vi "Replay AVI Movie.vi"() -> ()   [LabVIEW 2015]
panel:
  in  "Bin Iteration":i32
  in  "Frame Interval (ms)":u32=100
  in  "AVI File Name":path=path "Z:/1_20140213R_Edited.avi"
  in  "N Frame":i32=100
  out "Frame #":i32
  out "Bin Image":T1(plugin-control)
  out "Original Image":T1(plugin-control)
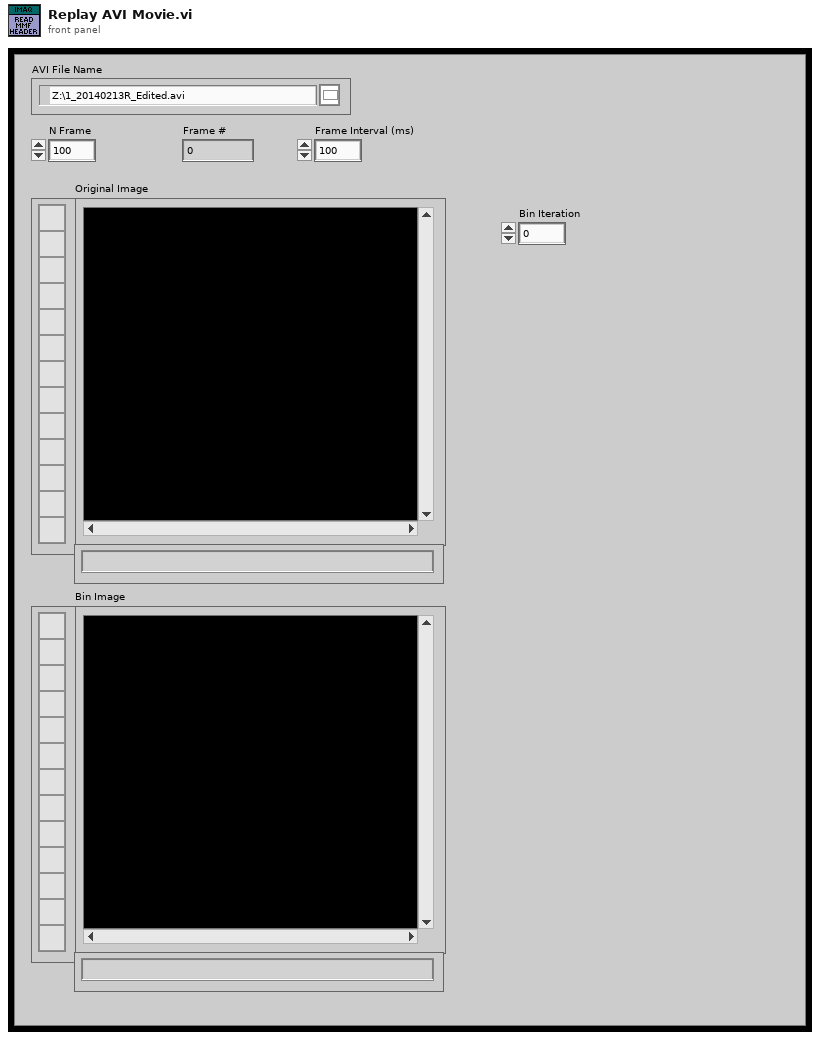
[diagram p1: front panel]
types:
  T1 = typedef "IMAQ Image.ctl" = refnum<image>
  T2 = typedef "IMAQ AVI2 Refnum.ctl" = refnum<k20>
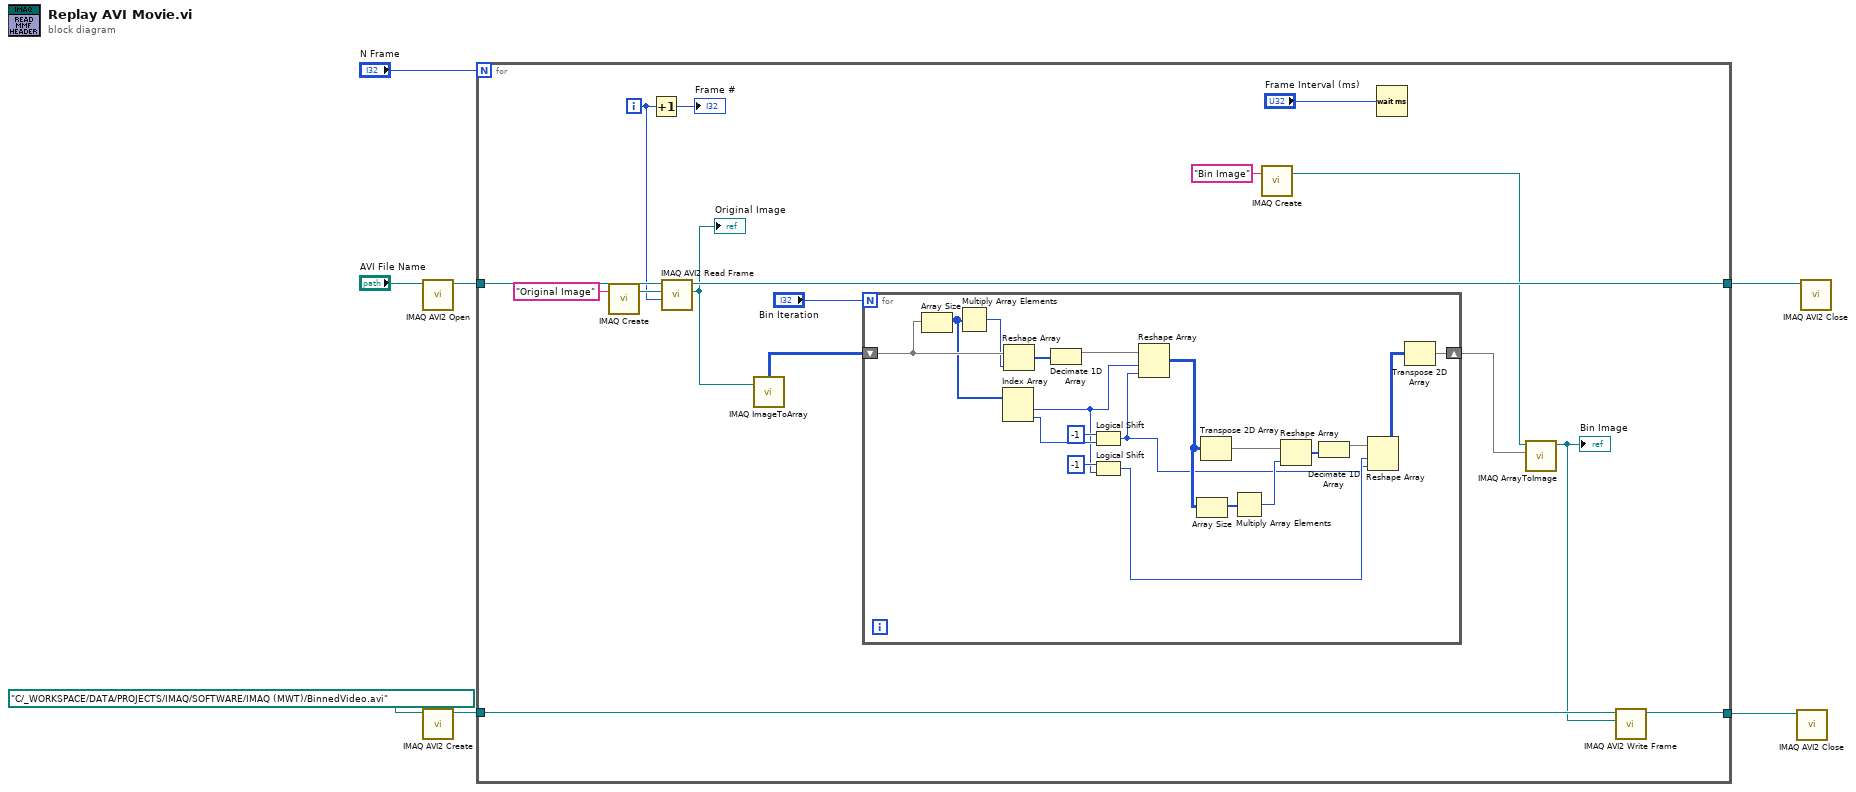
[diagram p0: block diagram]
diagram:
  n1 = call "IMAQ AVI2 Open"("AVI File Path"="AVI File Name") -> ("AVI Refnum"=w4:T2)  [unwired: 9 in, 1 out]
  n2 = call "IMAQ AVI2 Create"("AVI Path"=path "C:/_WORKSPACE/DATA/PROJECTS/IMAQ/SOFTWARE/IMAQ (MWT)/BinnedVideo.avi" ("AVI File Path")) -> ("AVI Refnum"=w2:T2)  [unwired: 9 in, 1 out]
  n3 = for {
    N: "N Frame" -> [_]
    tunnel: w4 -> [w22]
    tunnel: [w21] -> w7
    tunnel: w2 -> [w10]
    tunnel: [w9] -> w1
    i -> [w12]
    n4 = call "IMAQ Create"("Image Name"="Original Image") -> ("New Image"=w13:T1)  [unwired: 4 in, 1 out]
    n5 = Increment(x=w12) -> (x+1=→"Frame #":i32)
    n6 = call "IMAQ AVI2 Read Frame"("Frame Number"=w12, "Image"=w13, "AVI Refnum"=w22) -> ("Image Out"=w18:T1, "AVI Refnum (duplicate)"=w21:T2)  [unwired: 6 in, 1 out]
    "Original Image" <- w18
    n7 = call "IMAQ ImageToArray"("Image"=w18) -> ("Image Pixels (U8)"=w17:u8[][])  [unwired: 3 in, 4 out]
    n8 = for {
      N: "Bin Iteration" -> [_]
      shift-right: [w24] -> w16
      shift-left: w17 -> [w42]
      n9 = Array Size(array=w42) -> (size(s)=w39:i32[])
      n10 = Multiply Array Elements(1:w39) -> (0:w41:i32)
      n11 = Index Array(array=w39) -> (element #1=w30:i32, element #2=w38:i32)  [unwired: 2 in]
      n12 = Reshape Array(w42, w41) -> (w40:u8[])
      n13 = Decimate 1D Array(w40) -> (w26:u8[])  [unwired: 1 out]
      n14 = Logical Shift(y=i16 -1, x=w38) -> (x << y=w28:i32)
      n15 = Logical Shift(y=i16 -1, x=w30) -> (x << y=w29:i32)
      n16 = Reshape Array(w26, w30, w28) -> (w34:u8[][])
      n17 = Array Size(array=w34) -> (size(s)=w35:i32[])
      n18 = Transpose 2D Array(2D array=w34) -> (transposed array=w36:u8[][])
      n19 = Multiply Array Elements(1:w35) -> (0:w33:i32)
      n20 = Reshape Array(w36, w33) -> (w32:u8[])
      n21 = Decimate 1D Array(w32) -> (w25:u8[])  [unwired: 1 out]
      n22 = Reshape Array(w25, w29, w28) -> (w27:u8[][])
      n23 = Transpose 2D Array(2D array=w27) -> (transposed array=w24:u8[][])
    }
    n24 = call "IMAQ Create"("Image Name"="Bin Image") -> ("New Image"=w15:T1)  [unwired: 4 in, 1 out]
    n25 = Wait (ms)(milliseconds to wait="Frame Interval (ms)") -> ()  [unwired: 1 out]
    n26 = call "IMAQ ArrayToImage"("Image Pixels (U8)"=w16, "Image"=w15) -> ("Image Out"=w8:T1)  [unwired: 8 in, 1 out]
    "Bin Image" <- w8
    n27 = call "IMAQ AVI2 Write Frame"("Image"=w8, "AVI Refnum"=w10) -> ("AVI Refnum (duplicate)"=w9:T2)  [unwired: 7 in, 2 out]
  }
  n28 = call "IMAQ AVI2 Close"("AVI Refnum"=w1) -> ()  [unwired: 10 in, 1 out]
  n29 = call "IMAQ AVI2 Close"("AVI Refnum"=w7) -> ()  [unwired: 10 in, 1 out]
